vi "Wise Drive.vi"(1 "Joystick Control":dbl) -> (0 "Throttle":dbl)   [LabVIEW 2016]
panel:
  in  "Low slope":dbl=0.5
  in  "Switch value":dbl=0.7
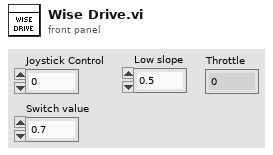
[diagram p1: front panel]
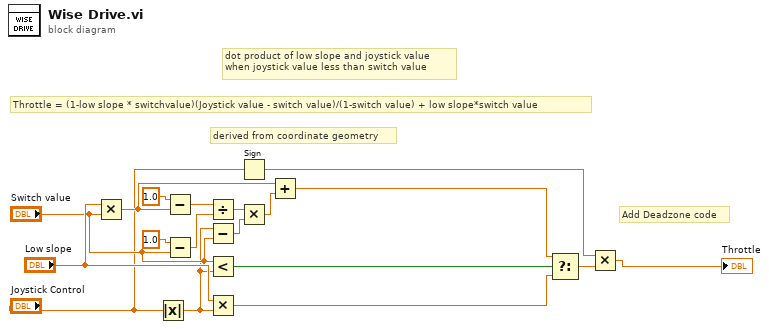
[diagram p0: block diagram]
diagram:
  # "Add Deadzone code"
  # "derived from coordinate geometry"
  # "Throttle = (1-low slope * switchvalue)(Joystick value - switch value)/(1-switch value) + low slope*switch value"
  # "dot product of low slope and joystick value \nwhen joystick value less than switch value"
  n1 = Multiply(x="Low slope", y="Switch value") -> (x*y=w14:dbl)
  n2 = Absolute Value(x="Joystick Control") -> (abs(x)=w5:dbl)
  n3 = Subtract(x=1.0, y=w14) -> (x-y=w13:dbl)
  n4 = Subtract(x=1.0, y="Switch value") -> (x-y=w11:dbl)
  n5 = Divide(x=w13, y=w11) -> (x/y=w10:dbl)
  n6 = Subtract(x=w5, y="Switch value") -> (x-y=w9:dbl)
  n7 = Less?(x="Switch value", y=w5) -> (x < y?=w17:bool)
  n8 = Multiply(x="Low slope", y=w5) -> (x*y=w18:dbl)
  n9 = Sign(1:"Joystick Control") -> (0:w4:dbl)
  n10 = Multiply(x=w10, y=w9) -> (x*y=w8:dbl)
  n11 = Add(x=w14, y=w8) -> (x+y=w16:dbl)
  n12 = Select(t=w16, s=w17, f=w18) -> (s? t:f=w3:dbl)
  n13 = Multiply(x=w4, y=w3) -> (x*y=→"Throttle":dbl)
